vi "test - Find Disable Structure valid.vi"(8 "error in (no error)":errorcluster, 11 "TestCase in":refnum<class "Find Disable Structure.lvclass">) -> (0 "error out":errorcluster, 3 "TestCase out":refnum<class "Find Disable Structure.lvclass">)   [LabVIEW 2018, in "Find Disable Structure.lvclass"]
uses:
  Find Disable Structure.lvclass
  <vilib>/addons/_JKI Toolkits/VI Tester/TestCase.llb/TestCase.lvclass
  C:/Program Files (x86)/National Instruments/LabVIEW 2018/vi.lib/addons/_JKI Toolkits/VI Tester/TestCase.llb/TestCase.lvclass
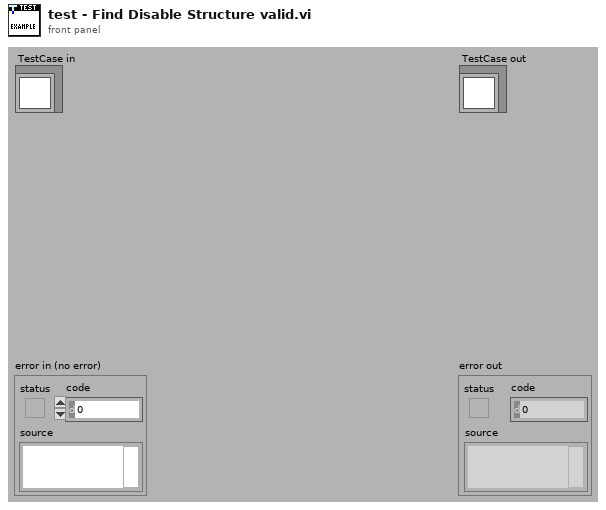
[diagram p1: front panel]
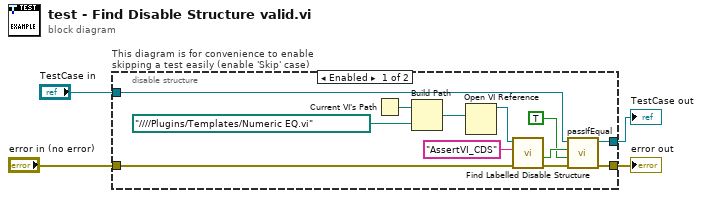
[diagram p0: block diagram]
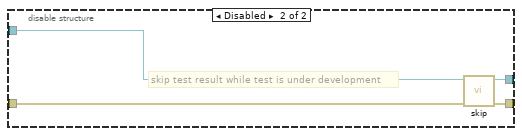
[diagram p2: hidden frame]
diagram:
  n1 = disable-structure "This diagram is for convenience to enable skipping a test easily (enable 'Skip' case)" shown="Enabled" {
    disable-tunnel: "TestCase in" -> [w8 w20]
    disable-tunnel: [w16 w18] -> w1
    disable-tunnel: [w15 w19] -> w3
    disable-tunnel: "error in (no error)" -> [w14 w17]
    frame Enabled {
      n2 = Current VI's Path() -> (path=w7:path)
      n3 = Build Path(base path=w7, name or relative path=path "../../../../Plugins/Templates/Numeric EQ.vi" ("vi path")) -> (appended path=w5:path)
      n4 = Open VI Reference(vi path=w5) -> (vi reference=w13:refnum<vi>)  [unwired: 5 in, 1 out]
      n5 = call "Find Labelled Disable Structure.vi"("error in (no error)"=w14, "Label"="AssertVI_CDS", "VI in"=w13) -> ("error out"=w9:errorcluster, "Found?"=w11:bool)  [unwired: 6 in, 1 out]
      n6 = call-dynamic "passIfEqual.vi"("error in (no error)"=w9, "y"=TRUE, "x"=w11, "TestCase in"=w8) -> ("error out"=w15:errorcluster, "TestCase out"=w16:refnum<class "Find Disable Structure.lvclass">)  [unwired: 6 in]
    }
    frame Disabled {
      # "skip test result while test is under development"
      n7 = call <vilib>:"skip.vi"("error in (no error)"=w17, "TestCase in"=w20) -> ("error out"=w19:errorcluster, "TestCase out"=w18:refnum<class "Find Disable Structure.lvclass">)  [unwired: 8 in]
    }
  }
  "error out" <- w3
  "TestCase out" <- w1
